vi "ConvertPB_LongDelay.vi"(0 "PB VLIW Array in":T2(array[cluster]) {"Output Bits" format="%x"}, 1 "Definitions":T1={"External MemorySize"=32768, "Internal Memory Size"=512, "Overhead Ticks"=3, "Min Delay Loops"=3, "Loop Count Correction"=1, "Long Delay Loop Count Correction"=2, "Min Instruction Ticks"=6, "Long Delay Ticks"=4294967295, "Clock Period (s)"=1e-08, "Overhead Time (s)"=3e-08, "Min Instruction Cycle Time (s)"=9e-08, "Long Delay Time (s) "=42.94967298} {"Long Delay Time (s)" format="%.8p"; "Min Instruction Cycle Time (s)" format="%.0p"; "Overhead Time (s)" format="%.0p"; "Clock Period (s)" format="%.0p"; "Long Delay Ticks" format="%.0x"}, 2 "error in (no error)":errorcluster, 3 "Full trigger mask":u32 format="%x") -> (5 "PB VLIW Array out":T2(array[cluster]) {"Output Bits" format="%x"}, 6 "error out":errorcluster)   [LabVIEW 2013, in "PulseBlaster.lvlib"]
doc: "Accounts for the strange clocking in of the line following a trigger while the PB is waiting for an external analog trigger."
uses:
  PulseBlaster.lvlib
panel:
  # "(Period*Long D Ticks)+Overhead time"
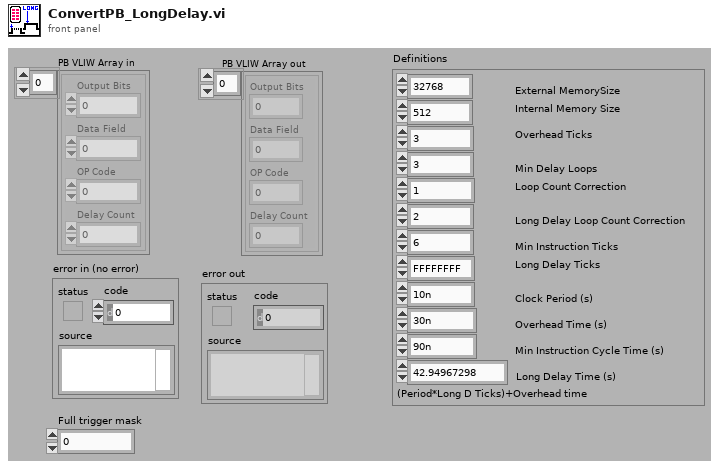
[diagram p1: front panel]
types:
  T1 = cluster{"External MemorySize":u16, "Internal Memory Size":u16, "Overhead Ticks":u8, "Min Delay Loops":u8, "Loop Count Correction":u8, "Long Delay Loop Count Correction":u8, "Min Instruction Ticks":u8, "Long Delay Ticks":u64, "Clock Period (s)":dbl, "Overhead Time (s)":dbl, "Min Instruction Cycle Time (s)":dbl, "Long Delay Time (s) ":dbl}
  T2 = cluster{"Output Bits":u32, "Data Field":u32, "OP Code":u8, "Delay Count":u64}[]
  T3 = cluster{"Output Bits":u32, "Data Field":u32, "OP Code":u8, "Delay Count":u32}[]
  T4 = cluster{"Output Bits":u32, "Data Field":u32, "OP Code":u8, u32}
  T5 = cluster{"Output Bits":u32, "Data Field":u32, "OP Code":u8, "Delay Count":u64}
  T6 = cluster{"Output Bits":u32, u32, "OP Code":u8, "Delay Count":u64}
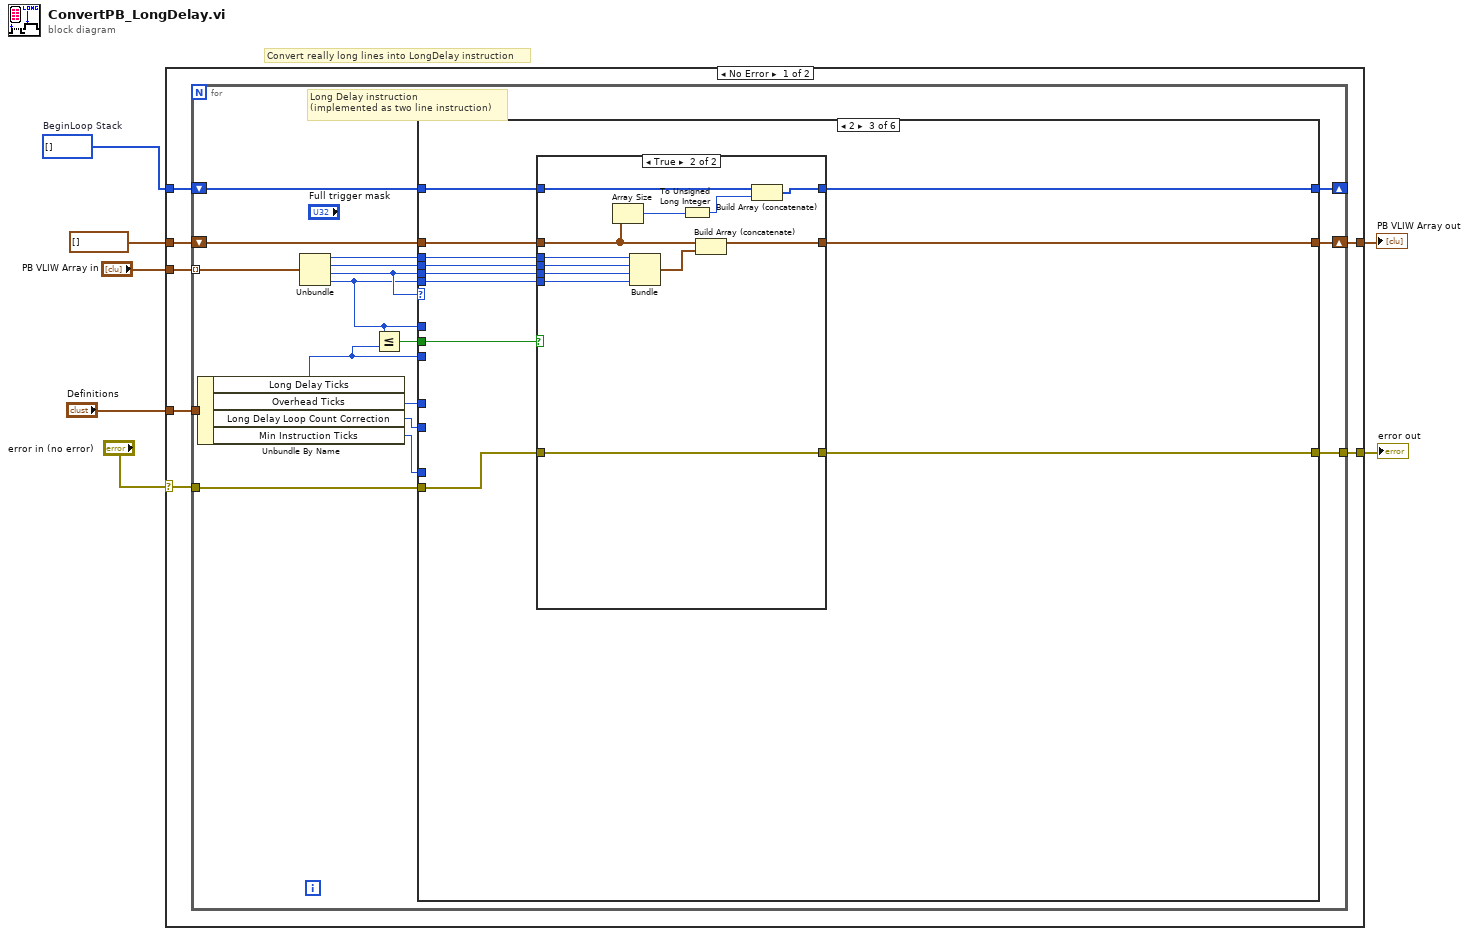
[diagram p0: block diagram]
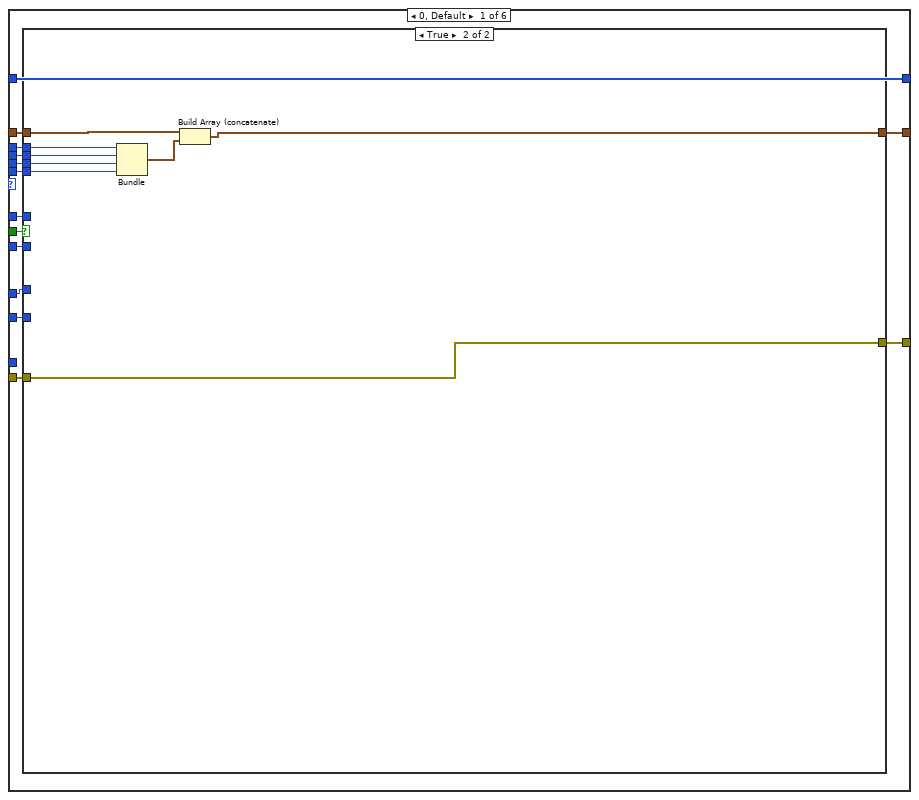
[diagram p2: hidden frame]
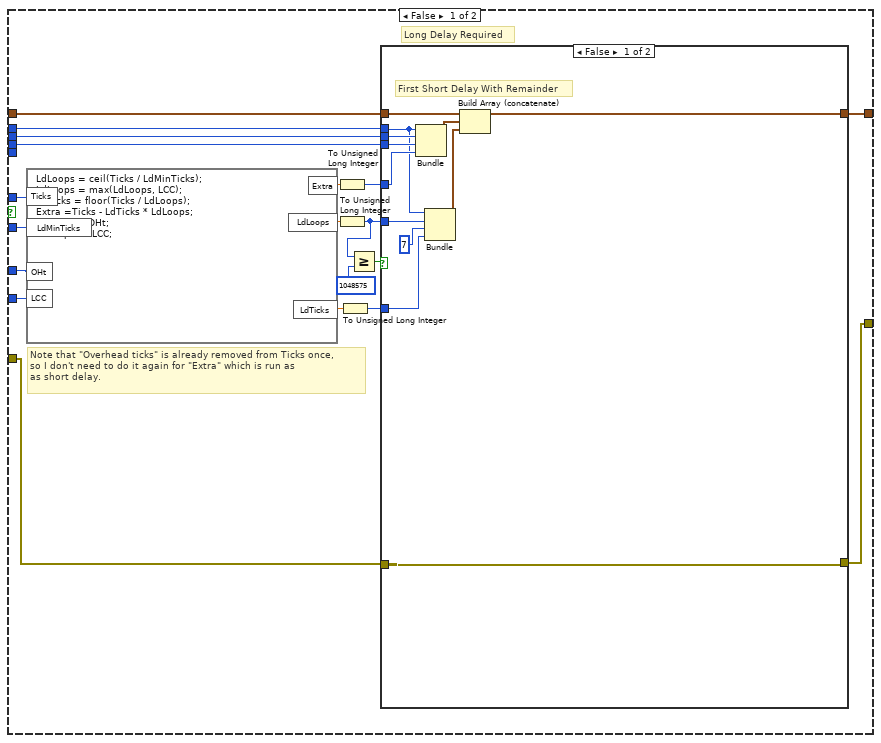
[diagram p3: hidden frame]
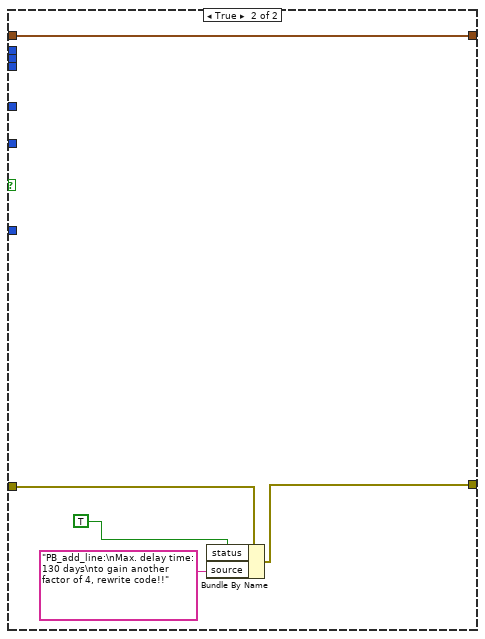
[diagram p4: hidden frame]
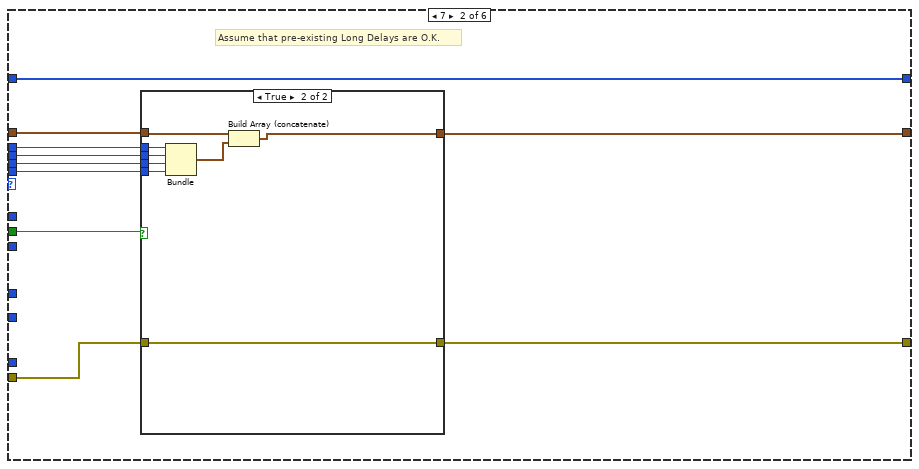
[diagram p5: hidden frame]
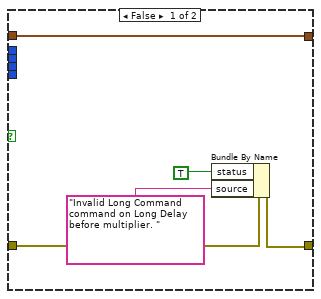
[diagram p6: hidden frame]
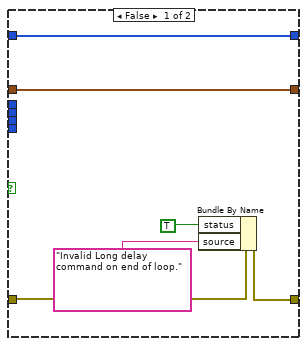
[diagram p7: hidden frame]
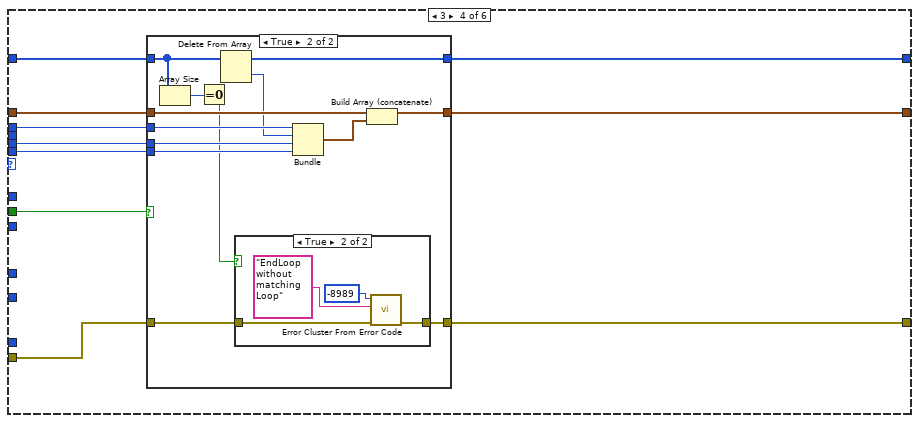
[diagram p8: hidden frame]
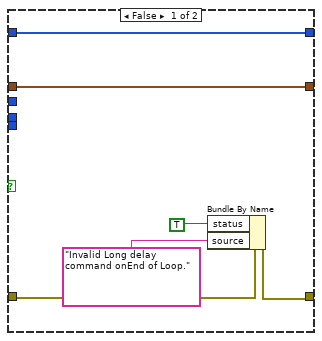
[diagram p9: hidden frame]
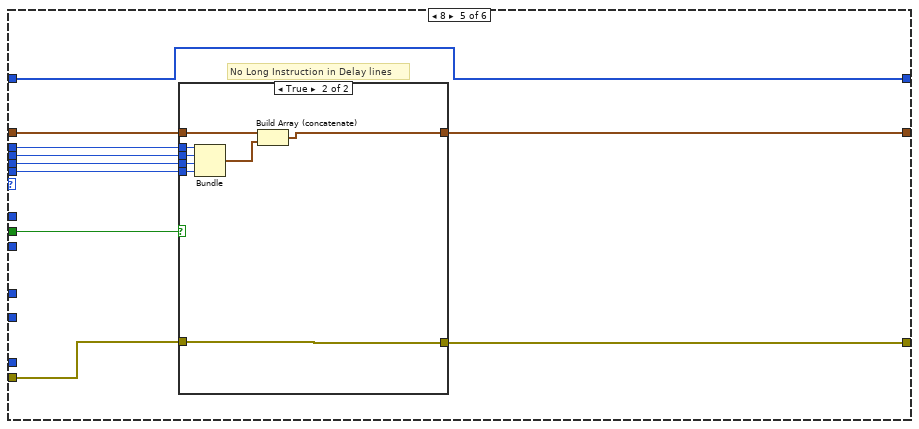
[diagram p11: hidden frame]
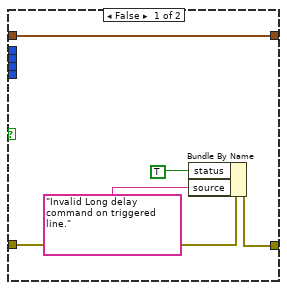
[diagram p12: hidden frame]
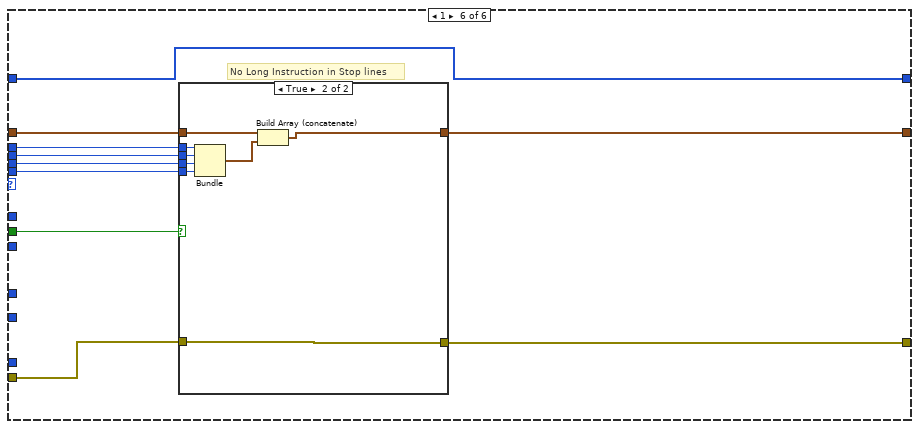
[diagram p13: hidden frame]
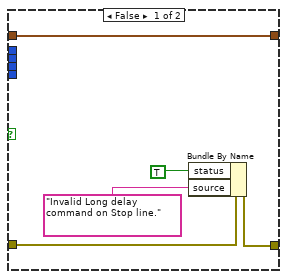
[diagram p14: hidden frame]
diagram:
  w1 = u32[] []  # BeginLoop Stack
  # "Convert really long lines into LongDelay instruction"
  n1 = case shown="No Error" "error in (no error)" {
    selector: "error in (no error)" -> [w10 w222]
    tunnel: T3 [] -> [w14 _]
    tunnel: [w13 w223] -> w6
    tunnel: "PB VLIW Array in" -> [w12 w223]
    tunnel: [w11 w222] -> w4
    tunnel: "Definitions" -> [w9 _]
    tunnel: w1 -> [w8 _]
    frame No Error {
      n2 = for {
        tunnel: w12 -> [w31] mode=indexing
        shift-right: [w26] -> w13
        shift-left: w14 -> [w29]
        tunnel: w10 -> [w28]
        tunnel: [w27] -> w11
        tunnel: w9 -> [w21]
        shift-right: [w16] -> _
        shift-left: w8 -> [w15]
        # "Long Delay instruction \n(implemented as two line instruction)"
        n3 = Unbundle By Name(w21) -> ("Long Delay Ticks"=w17:u64, "Overhead Ticks"=w18:u8, "Long Delay Loop Count Correction"=w19:u8, "Min Instruction Ticks"=w20:u8)
        n4 = Unbundle(w31) -> ("Output Bits"=w24:u32, "Data Field"=w30:u32, "OP Code"=w25:u8, "Delay Count"=w22:u64)
        n5 = Less Or Equal?(x=w22, y=w17) -> (x <= y?=w23:bool)
        n6 = case shown="2" w25 {
          tunnel: w30 -> [w39 w93 w123 _ w179 w202]
          tunnel: w25 -> [w38 w92 w122 w151 w178 w201]
          tunnel: w22 -> [w37 w91 w121 w150 w177 w200]
          tunnel: w29 -> [w45 w99 w118 w149 w185 w208]
          tunnel: w28 -> [w42 w97 w117 w146 w184 w207]
          tunnel: [w41 w96 w116 w145 w183 w206] -> w27
          tunnel: w18 -> [w34 _ _ _ _ _]
          tunnel: w20 -> [_ _ _ _ _ _]
          tunnel: w24 -> [w40 w94 w120 w148 w180 w203]
          tunnel: [w44 w98 w119 w147 w182 w205] -> w26
          tunnel: w23 -> [w43 w95 w115 w144 w181 w204]
          tunnel: w22 -> [w36 _ _ _ _ _]
          tunnel: w17 -> [w35 _ _ _ _ _]
          tunnel: w19 -> [w33 _ _ _ _ _]
          tunnel: [w32 w90 w114 w142 w176 w199] -> w16
          tunnel: w15 -> [w32 w90 w113 w143 w176 w199]
          frame 0, Default {
            n7 = case shown="True" w43 {
              tunnel: w45 -> [w60 w87]
              tunnel: [w59 w86] -> w44
              tunnel: w42 -> [w62 w89]
              tunnel: [w61 w89] -> w41
              tunnel: w40 -> [w55 w85]
              tunnel: w39 -> [w54 w84]
              tunnel: w38 -> [w53 w83]
              tunnel: w37 -> [_ w82]
              tunnel: w36 -> [w63 _]
              tunnel: w35 -> [w64 _]
              tunnel: w34 -> [w47 _]
              tunnel: w33 -> [w46 _]
              frame False {
                # "Note that \"Overhead ticks\" is already removed from Ticks once,\nso I don't need to do it again for \"Extra\" which is run as \nas short delay."
                # "Long Delay Required"
                n8 = formula code="LdLoops = ceil(Ticks / LdMinTicks);\nLdLoops = max(LdLoops, LCC);\nLdTicks = floor(Ticks / LdLoops);\nExtra =Ticks - LdTicks * LdLoops;\nLdTicks -= OHt;\nLdLoops -= LCC;"("LdMinTicks"=w64, "Ticks"=w63, "OHt"=w47, "LCC"=w46) -> ("LdLoops"=w49:dbl, "LdTicks"=w51:dbl, "Extra"=w56:dbl)
                n9 = To Unsigned Long Integer(number=w56) -> (unsigned 32bit integer=w52:u32)
                n10 = To Unsigned Long Integer(number=w49) -> (unsigned 32bit integer=w48:u32)
                n11 = To Unsigned Long Integer(number=w51) -> (unsigned 32bit integer=w50:u32)
                n12 = Greater Or Equal?(x=w48, y=1048575) -> (x >= y?=w58:bool)
                n13 = case shown="False" w58 {
                  tunnel: w62 -> [w76 w79]
                  tunnel: [w76 w78] -> w61
                  tunnel: w60 -> [w72 w77]
                  tunnel: [w70 w77] -> w59
                  tunnel: w52 -> [w71 _]
                  tunnel: w55 -> [w68 _]
                  tunnel: w54 -> [w75 _]
                  tunnel: w53 -> [w74 _]
                  tunnel: w50 -> [w66 _]
                  tunnel: w48 -> [w67 _]
                  frame False {
                    # "First Short Delay With Remainder"
                    n14 = Bundle("Output Bits"=w68, "Data Field"=w75, "OP Code"=w74, w71) -> (w73:T4)  [unwired: 1 out]
                    n15 = Bundle("Output Bits"=w68, w67, u8 7, w66) -> (w65:cluster{"Output Bits":u32, u32, u8, u32})  [unwired: 1 out]
                    n16 = Build Array (concatenate)(w72, w73, w65) -> (w70:T2)
                  }
                  frame True {
                    n17 = Bundle By Name(cluster=w79, "status"=TRUE, "source"="PB_add_line:\nMax. delay time: 130 days\nto gain another factor of 4, rewrite code!!") -> (w78:errorcluster)
                  }
                }
              }
              frame True {
                n18 = Bundle("Output Bits"=w85, "Data Field"=w84, "OP Code"=w83, "Delay Count"=w82) -> (w88:T5)  [unwired: 1 out]
                n19 = Build Array (concatenate)(w87, w88) -> (w86:T2)
              }
            }
          }
          frame 7 {
            # "Assume that pre-existing Long Delays are O.K."
            n20 = case shown="True" w95 {
              tunnel: w99 -> [w104 w110]
              tunnel: [w104 w109] -> w98
              tunnel: w97 -> [w101 w112]
              tunnel: [w100 w112] -> w96
              tunnel: w94 -> [_ w108]
              tunnel: w93 -> [_ w107]
              tunnel: w92 -> [_ w106]
              tunnel: w91 -> [_ w105]
              frame False {
                n21 = Bundle By Name(cluster=w101, "status"=TRUE, "source"="Invalid Long Command  command on Long Delay before multiplier. ") -> (w100:errorcluster)
              }
              frame True {
                n22 = Bundle("Output Bits"=w108, "Data Field"=w107, "OP Code"=w106, "Delay Count"=w105) -> (w111:T5)  [unwired: 1 out]
                n23 = Build Array (concatenate)(w110, w111) -> (w109:T2)
              }
            }
          }
          frame 2 {
            n24 = case shown="True" w115 {
              tunnel: w123 -> [_ w141]
              tunnel: w122 -> [_ w140]
              tunnel: w121 -> [_ w139]
              tunnel: w120 -> [_ w138]
              tunnel: [w125 w137] -> w119
              tunnel: w118 -> [w125 w135]
              tunnel: w117 -> [w127 w134]
              tunnel: [w126 w134] -> w116
              tunnel: [w124 w131] -> w114
              tunnel: w113 -> [w124 w132]
              frame False {
                n25 = Bundle By Name(cluster=w127, "status"=TRUE, "source"="Invalid Long delay command on end of loop.") -> (w126:errorcluster)
              }
              frame True {
                n26 = Array Size(array=w135) -> (size(s)=w130:i32)
                n27 = Bundle("Output Bits"=w138, "Data Field"=w141, "OP Code"=w140, "Delay Count"=w139) -> (w136:T5)  [unwired: 1 out]
                n28 = To Unsigned Long Integer(number=w130) -> (unsigned 32bit integer=w133:u32)
                n29 = Build Array (concatenate)(w135, w136) -> (w137:T2)
                n30 = Build Array (concatenate)(w132, w133) -> (w131:u32[])
              }
            }
          }
          frame 3 {
            n31 = case shown="True" w144 {
              tunnel: w151 -> [_ w170]
              tunnel: w150 -> [_ w169]
              tunnel: w149 -> [w153 w168]
              tunnel: w148 -> [_ w167]
              tunnel: [w153 w166] -> w147
              tunnel: w146 -> [w155 w162]
              tunnel: [w154 w161] -> w145
              tunnel: w143 -> [w152 w159]
              tunnel: [w152 w164] -> w142
              frame False {
                n32 = Bundle By Name(cluster=w155, "status"=TRUE, "source"="Invalid Long delay command onEnd of Loop.") -> (w154:errorcluster)
              }
              frame True {
                n33 = Array Size(array=w159) -> (size(s)=w160:i32)
                n34 = Equal To 0?(x=w160) -> (x = 0?=w158:bool)
                n35 = Delete From Array(array=w159) -> (deleted portion=w163:u32, array with subset deleted=w164:u32[])  [unwired: 2 in]
                n36 = case shown="True" w158 {
                  tunnel: w162 -> [w171 w173]
                  tunnel: [w171 w172] -> w161
                  frame False {
                  }
                  frame True {
                    n37 = call <vilib>:"Error Cluster From Error Code.vi"("error in (no error)"=w173, "error message (\"\")"="EndLoop without matching Loop" ("error message (\"\")"), "error code (0)"=-8989) -> ("error out"=w172:errorcluster)  [unwired: 6 in]
                  }
                }
                n38 = Bundle("Output Bits"=w167, w163, "OP Code"=w170, "Delay Count"=w169) -> (w165:T6)  [unwired: 1 out]
                n39 = Build Array (concatenate)(w168, w165) -> (w166:T2)
              }
            }
          }
          frame 8 {
            # "No Long Instruction in Delay lines"
            n40 = case shown="True" w181 {
              tunnel: w185 -> [w186 w193]
              tunnel: w184 -> [w190 w198]
              tunnel: [w189 w198] -> w183
              tunnel: [w186 w192] -> w182
              tunnel: w180 -> [_ w197]
              tunnel: w179 -> [_ w196]
              tunnel: w178 -> [_ w195]
              tunnel: w177 -> [_ w194]
              frame False {
                n41 = Bundle By Name(cluster=w190, "status"=TRUE, "source"="Invalid Long delay command on triggered line.") -> (w189:errorcluster)
              }
              frame True {
                n42 = Bundle("Output Bits"=w197, "Data Field"=w196, "OP Code"=w195, "Delay Count"=w194) -> (w191:T5)  [unwired: 1 out]
                n43 = Build Array (concatenate)(w193, w191) -> (w192:T2)
              }
            }
          }
          frame 1 {
            # "No Long Instruction in Stop lines"
            n44 = case shown="True" w204 {
              tunnel: w208 -> [w209 w216]
              tunnel: w207 -> [w213 w221]
              tunnel: [w212 w221] -> w206
              tunnel: [w209 w215] -> w205
              tunnel: w203 -> [_ w220]
              tunnel: w202 -> [_ w219]
              tunnel: w201 -> [_ w218]
              tunnel: w200 -> [_ w217]
              frame False {
                n45 = Bundle By Name(cluster=w213, "status"=TRUE, "source"="Invalid Long delay command on Stop line.") -> (w212:errorcluster)
              }
              frame True {
                n46 = Bundle("Output Bits"=w220, "Data Field"=w219, "OP Code"=w218, "Delay Count"=w217) -> (w214:T5)  [unwired: 1 out]
                n47 = Build Array (concatenate)(w216, w214) -> (w215:T2)
              }
            }
          }
        }
      }
    }
    frame Error {
    }
  }
  "error out" <- w4
  "PB VLIW Array out" <- w6
